vi "Word_Bookmark_Table_Exists.vi"(0 "report in":refnum<class "NI_report.lvclass">, 1 "MS Office parameters":T1, 9 "get table ref?":bool, 11 "error in (no error)":errorcluster) -> (4 "report out":refnum<class "NI_report.lvclass">, 6 "bookmark to existing table?":bool, 10 "table ref":refnum<k7>, 15 "error out":errorcluster)   [LabVIEW 2020, in "NI_Word.lvclass"]
uses:
  <vilib>/Utility/NIReport.llb/Word/NI_Word.lvclass
  <vilib>/Utility/NIReport.llb/NI_report.lvclass
  C:/Program Files (x86)/National Instruments/LabVIEW 2020/vi.lib/Utility/NIReport.llb/NI_report.lvclass
  <vilib>/Utility/NIReport.llb/Word/NI_Word.lvclass/NI_Word.ctl
  <vilib>/Utility/NIReport.llb/NI_ReportGenerationCore.lvlib
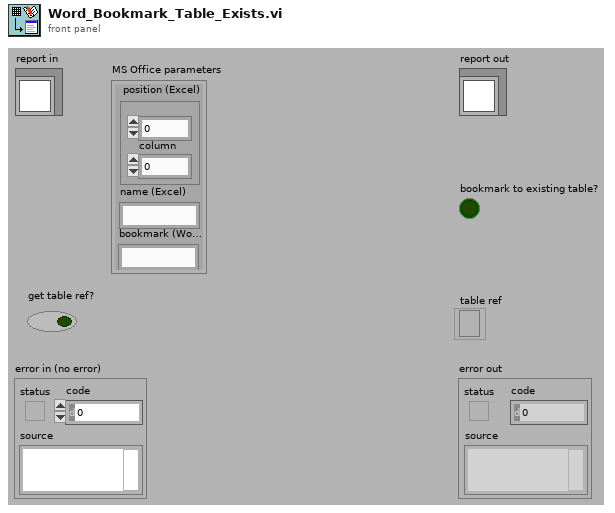
[diagram p1: front panel]
types:
  T1 = cluster{"position (Excel)":cluster{"row":i32, "column":i32}, "name (Excel) ":string, "bookmark (Word)":string}
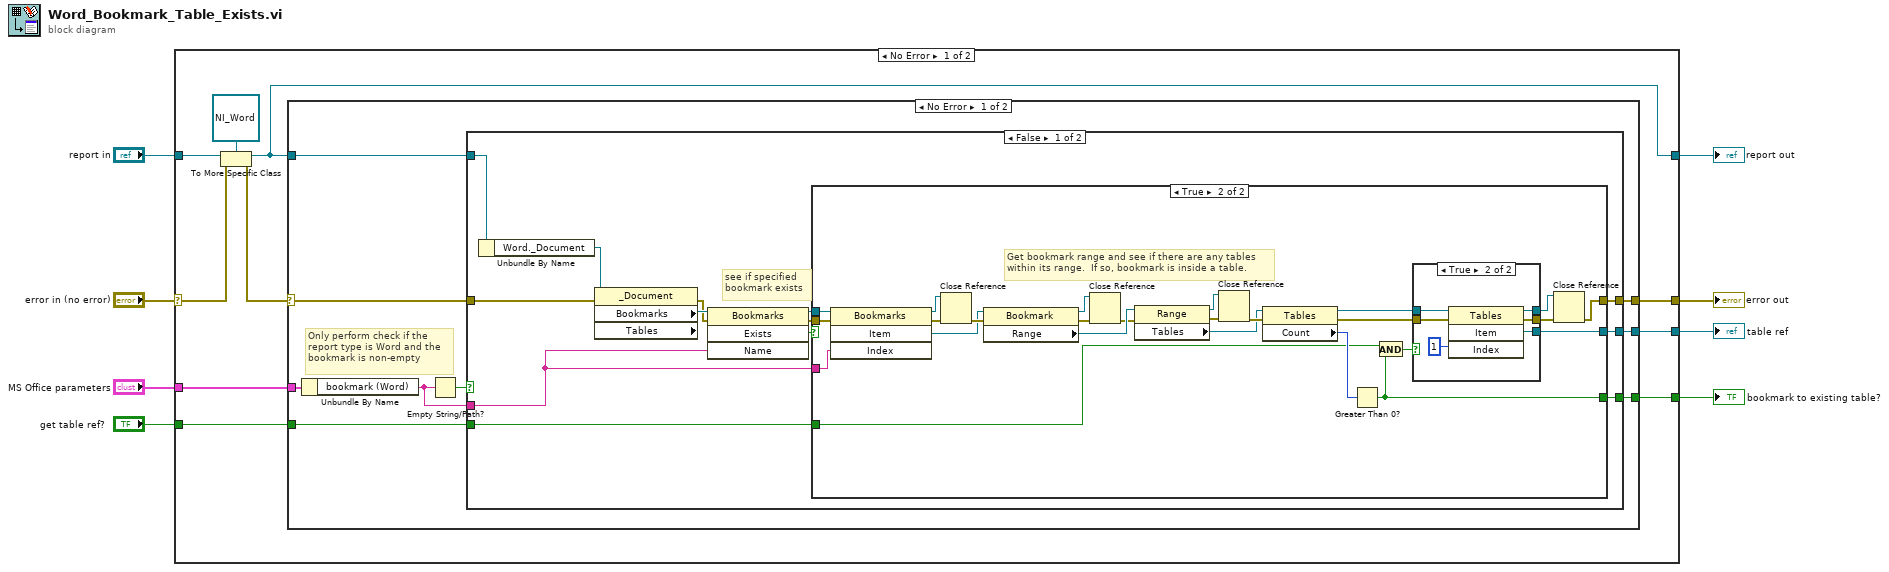
[diagram p0: block diagram]
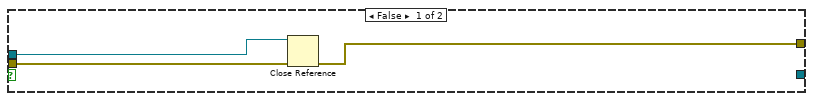
[diagram p2: hidden frame]
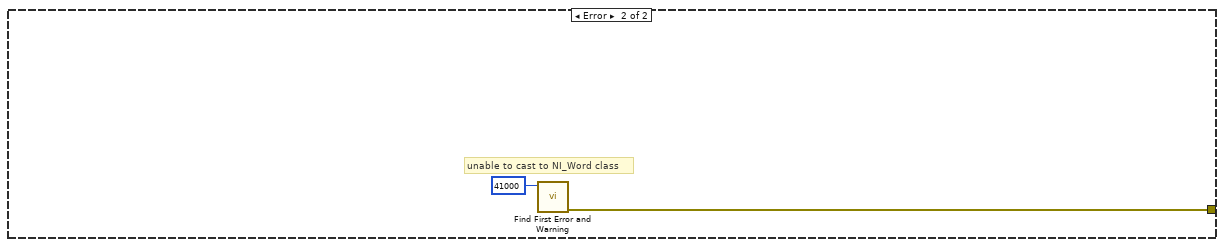
[diagram p5: hidden frame]
diagram:
  n1 = case shown="No Error" "error in (no error)" {
    selector: "error in (no error)" -> [w10 w81]
    tunnel: [w16 w81] -> w7
    tunnel: [w11 w80] -> w5
    tunnel: "report in" -> [w12 w80]
    tunnel: "get table ref?" -> [w18 _]
    tunnel: "MS Office parameters" -> [w17 _]
    tunnel: [w15 _] -> w2
    tunnel: [w14 _] -> w1
    frame No Error {
      n2 = To More Specific Class(target class=refnum<class "NI_Word.lvclass"> refnum ("report in"), reference=w12, error in=w10) -> (specific class reference=w11:refnum<class "NI_Word.lvclass">, error out=w9:errorcluster)
      n3 = case shown="No Error" w9 {
        selector: w9 -> [w19 _]
        tunnel: w18 -> [w26 _]
        tunnel: w17 -> [w25 _]
        tunnel: [w23 w78] -> w16
        tunnel: [w22 _] -> w15
        tunnel: [w21 _] -> w14
        tunnel: w11 -> [w20 _]
        frame No Error {
          # "Only perform check if the\nreport type is Word and the\nbookmark is non-empty"
          n4 = Unbundle By Name(w25) -> ("bookmark (Word)"=w27:string)
          n5 = Empty String/Path?(string/path=w27) -> (empty?=w24:bool)
          n6 = case shown="False" w24 {
            tunnel: w19 -> [w29 w77]
            tunnel: [w34 w77] -> w23
            tunnel: [w37 _] -> w21
            tunnel: w27 -> [w35 _]
            tunnel: w26 -> [w32 _]
            tunnel: [w31 _] -> w22
            tunnel: w20 -> [w30 _]
            frame False {
              # "see if specified\nbookmark exists"
              n7 = Unbundle By Name(w30) -> ("Word._Document"=w28:refnum<k7>)
              n8 = property class="_Document" props=["Bookmarks", "Tables"](reference=w28, error in=w29) -> (error out=w33:errorcluster, "Bookmarks"=w40:refnum<k7>)  [unwired: 2 out]
              n9 = invoke class="Bookmarks" method="Exists"(reference=w40, error in=w33, "Name"=w35) -> (reference out=w36:refnum<k7>, error out=w39:errorcluster, "Exists"=w38:bool)  [unwired: 1 in, 1 out]
              n10 = case shown="True" w38 {
                tunnel: w39 -> [w43 w66]
                tunnel: [_ w45] -> w37
                tunnel: w36 -> [w42 w68]
                tunnel: w35 -> [_ w67]
                tunnel: [w41 w52] -> w34
                tunnel: w32 -> [_ w44]
                tunnel: [_ w47] -> w31
                frame False {
                  n11 = Close Reference(reference=w42, error in (no error)=w43) -> (error out=w41:errorcluster)
                }
                frame True {
                  # "Get bookmark range and see if there are any tables\nwithin its range.  If so, bookmark is inside a table."
                  n12 = invoke class="Bookmarks" method="Item"(reference=w68, error in=w66, "Index"=w67) -> (reference out=w64:refnum<k7>, error out=w65:errorcluster, "Item"=w62:refnum<k7>)  [unwired: 1 in, 1 out]
                  n13 = Close Reference(reference=w64, error in (no error)=w65) -> (error out=w63:errorcluster)
                  n14 = property class="Bookmark"(reference=w62, error in=w63) -> (reference out=w60:refnum<k7>, error out=w61:errorcluster, "Range"=w59:refnum<k7>)
                  n15 = Close Reference(reference=w60, error in (no error)=w61) -> (error out=w58:errorcluster)
                  n16 = property class="Range"(reference=w59, error in=w58) -> (reference out=w56:refnum<k7>, error out=w57:errorcluster, "Tables"=w53:refnum<k7>)
                  n17 = Close Reference(reference=w56, error in (no error)=w57) -> (error out=w55:errorcluster)
                  n18 = property class="Tables"(reference=w53, error in=w55) -> (reference out=w50:refnum<k7>, error out=w51:errorcluster, "Count"=w54:i32)
                  n19 = Greater Than 0?(x=w54) -> (x > 0?=w45:bool)
                  n20 = And(x=w44, y=w45) -> (x .and. y?=w46:bool)
                  n21 = case shown="True" w46 {
                    tunnel: w51 -> [w70 w76]
                    tunnel: w50 -> [w69 w75]
                    tunnel: [w70 w74] -> w49
                    tunnel: [w69 w73] -> w48
                    tunnel: [_ w72] -> w47
                    frame False {
                    }
                    frame True {
                      n22 = invoke class="Tables" method="Item"(reference=w75, error in=w76, "Index"=1) -> (reference out=w73:refnum<k7>, error out=w74:errorcluster, "Item"=w72:refnum<k7>)  [unwired: 1 in, 1 out]
                    }
                  }
                  n23 = Close Reference(reference=w48, error in (no error)=w49) -> (error out=w52:errorcluster)
                }
              }
            }
            frame True {
            }
          }
        }
        frame Error {
          # "unable to cast to NI_Word class"
          n24 = call <vilib>:"Find First Error and Warning.vi"("error code"=41000) -> ("error out"=w78:errorcluster)  [unwired: 2 in, 4 out]
        }
      }
    }
    frame Error {
    }
  }
  "error out" <- w7
  "report out" <- w5
  "bookmark to existing table?" <- w1
  "table ref" <- w2
